vi "Initialize Instrument Engine.vi"(8 "error in (no error)":errorcluster, 9 "Name":string, 11 "Process":refnum<class "Process.lvclass">) -> (0 "error out":errorcluster, 2 "notification":bool, 3 "State Variables":T1)   [LabVIEW 2023, in "Instrument Addon Engine.lvlib"]
uses:
  Instrument Addon Engine.lvlib
  Types/Engine State Variables.ctl
  <vilib>/NI/NI VeriStand Addon Network Comm/Engine/VeriStand Comm.lvclass
  <vilib>/NI/NIVS Inline Async API/_Data Access Engine/Data Access Engine/Types/Write.DVR.ctl
  <vilib>/NI/NIVS Inline Async API/_Data Access Engine/Access Type Classes/Write/Write.lvclass
  <vilib>/NI/NIVS Inline Async API/_Data Access Engine/Data Access Engine/Types/Read.DVR.ctl
  <vilib>/NI/NIVS Inline Async API/_Data Access Engine/Access Type Classes/Read/Read.lvclass
  <vilib>/NI/NIVS Inline Async API/_Data Access Engine/Data Access Engine/Types/ReadWrite.DVR.ctl
  <vilib>/NI/NIVS Inline Async API/_Data Access Engine/Access Type Classes/ReadWrite/ReadWrite.lvclass
  <vilib>/NI/NI VeriStand Addon Network Comm/Engine/VeriStand Comm.lvclass/VeriStand Comm.ctl
  <vilib>/NI/NIVS Inline Async API/_VS Inline Async API/Process/Process.lvclass/Process.ctl
  <vilib>/NI/NIVS Inline Async API/_VS Inline Async API/Error Handling Process/SubVIs/Error.ConvertArray.vi
  Addon Shared/SubVIs/Constants.vi
  <vilib>/Utility/SystemLogging/Write to System Log.vi
  <vilib>/NI/AMC/Create Message Queue.vi
  <vilib>/NI/STM/Connection Manager/TCP/Advanced/TCP Initialize Connection Manager (By Reference).vi
  <vilib>/NI/NIVS Inline Async API/_Data Access Engine/Data Access Engine/Methods/Write.Lookup.vi
  <vilib>/NI/NIVS Inline Async API/_Data Access Engine/Data Access Engine/Methods/Read.Lookup.vi
  <vilib>/NI/NIVS Inline Async API/_Data Access Engine/Data Access Engine/Methods/ReadWrite.Lookup.vi
  <vilib>/NI/NIVS Inline Async API/_Data Access Engine/Data Access Engine/Data Access Engine.lvclass
  Addon Shared/Instrument Addon Shared.lvlib
  <vilib>/NI/NIVS Inline Async API/_VS Inline Async API/Process/Process.lvclass
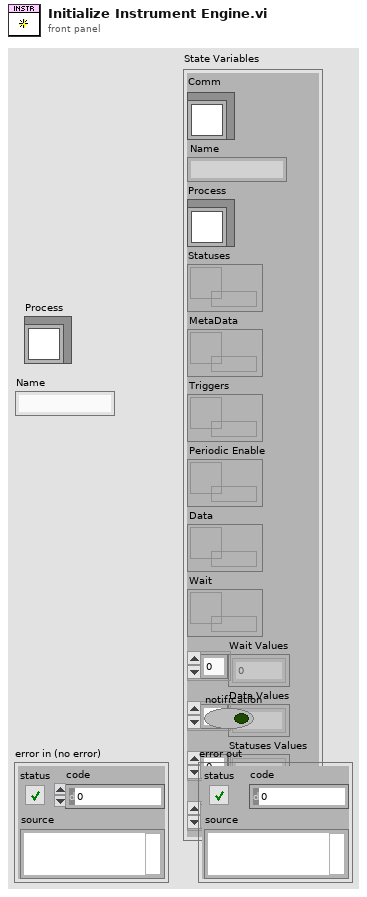
[diagram p1: front panel]
types:
  T1 = typedef "Instrument Addon Engine.lvlib/Engine State Variables.ctl" = cluster{"Comm":refnum<class "VeriStand Comm.lvclass">, "Name":string, "Process":refnum<class "Process.lvclass">, "Statuses":T2, "MetaData":T3, "Triggers":T4, "Periodic Enable":T3, "Data":T2, "Wait":T3, "Wait Values":dbl[], "Data Values":dbl[], "Statuses Values":dbl[], "MetaData Values":dbl[]}
  T2 = typedef "Data Access Engine.lvlib/Data Access Engine.lvclass/Write.DVR.ctl" = refnum<data-value>
  T3 = typedef "Data Access Engine.lvlib/Data Access Engine.lvclass/Read.DVR.ctl" = refnum<data-value>
  T4 = typedef "Data Access Engine.lvlib/Data Access Engine.lvclass/ReadWrite.DVR.ctl" = refnum<data-value>
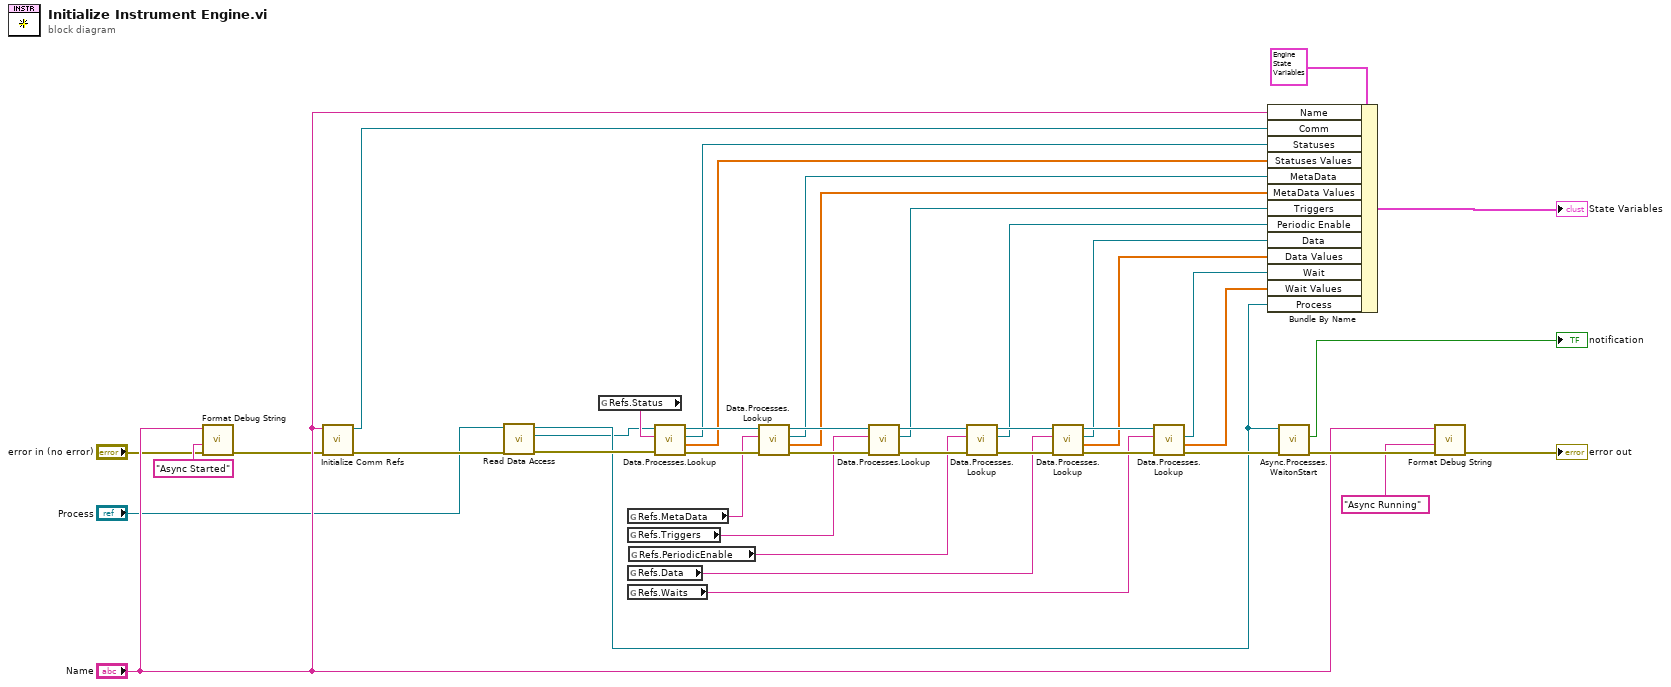
[diagram p0: block diagram]
diagram:
  n1 = call "Format Debug String.vi"("error in (no error)"="error in (no error)", "State"="Async Started" ("string"), "Name"="Name") -> ("error out"=w6:errorcluster)  [unwired: 7 in, 1 out]
  n2 = call <vilib>:"Initialize Comm Refs.vi"("error in (no error)"=w6, "Name"="Name") -> ("error out"=w5:errorcluster, "Comm.lvclass"=w42:refnum<class "VeriStand Comm.lvclass">)  [unwired: 8 in]
  n3 = call <vilib>:"Read Data Access.vi"("error in (no error)"=w5, "Process in"="Process") -> ("error out"=w4:errorcluster, "Data Access"=w1:refnum<class "Data Access Engine.lvclass">, "Process out"=w3:refnum<class "Process.lvclass">)  [unwired: 7 in]
  n4 = global read "Constants.vi" "Refs.Status"() -> (w24:string)
  n5 = global read "Constants.vi" "Refs.MetaData"() -> (w23:string)
  n6 = global read "Constants.vi" "Refs.Triggers"() -> (w21:string)
  n7 = global read "Constants.vi" "Refs.Data"() -> (w19:string)
  n8 = global read "Constants.vi" "Refs.Waits"() -> (w18:string)
  n9 = global read "Constants.vi" "Refs.PeriodicEnable"() -> (w20:string)
  n10 = call-poly <vilib>:"Data.Processes.Lookup.vi"("error in (no error)"=w4, "Name"=w24, "Data Access API in"=w1) -> ("error out"=w25:errorcluster, "Initial Values"=w15:dbl[], "Ref"=w13:T2, "Data Access API out"=w39:refnum<class "Data Access Engine.lvclass">)  [unwired: 5 in]
  n11 = call-poly <vilib>:"Data.Processes.Lookup.vi"("error in (no error)"=w25, "Name"=w23, "Data Access API in"=w39) -> ("error out"=w22:errorcluster, "Initial Values"=w16:dbl[], "Ref"=w26:T3, "Data Access API out"=w38:refnum<class "Data Access Engine.lvclass">)  [unwired: 5 in]
  n12 = call-poly <vilib>:"Data.Processes.Lookup.vi"("error in (no error)"=w22, "Name"=w21, "Data Access API in"=w38) -> ("error out"=w28:errorcluster, "Ref"=w27:T4, "Data Access API out"=w37:refnum<class "Data Access Engine.lvclass">)  [unwired: 5 in, 1 out]
  n13 = call-poly <vilib>:"Data.Processes.Lookup.vi"("error in (no error)"=w28, "Name"=w20, "Data Access API in"=w37) -> ("error out"=w29:errorcluster, "Ref"=w30:T3, "Data Access API out"=w36:refnum<class "Data Access Engine.lvclass">)  [unwired: 5 in, 1 out]
  n14 = call-poly <vilib>:"Data.Processes.Lookup.vi"("error in (no error)"=w29, "Name"=w19, "Data Access API in"=w36) -> ("error out"=w31:errorcluster, "Initial Values"=w14:dbl[], "Ref"=w32:T2, "Data Access API out"=w35:refnum<class "Data Access Engine.lvclass">)  [unwired: 5 in]
  n15 = call-poly <vilib>:"Data.Processes.Lookup.vi"("error in (no error)"=w31, "Name"=w18, "Data Access API in"=w35) -> ("error out"=w34:errorcluster, "Initial Values"=w17:dbl[], "Ref"=w33:T3)  [unwired: 5 in, 1 out]
  n16 = Bundle By Name(cluster=T1 {"Comm"=refnum, "Name"="", "Process"=refnum, "Statuses"=refnum, "MetaData"=refnum, "Triggers"=refnum, "Periodic Enable"=refnum, "Data"=refnum, "Wait"=refnum, "Wait Values"=[], "Data Values"=[], "Statuses Values"=[], "MetaData Values"=[]} ("State Variables"), "Name"="Name", "Comm"=w42, "Statuses"=w13, "Statuses Values"=w15, "MetaData"=w26, "MetaData Values"=w16, "Triggers"=w27, "Periodic Enable"=w30, "Data"=w32, "Data Values"=w14, "Wait"=w33, "Wait Values"=w17, "Process"=w3) -> (→"State Variables":T1)
  n17 = call <vilib>:"Async.Processes.WaitonStart.vi"("error in (no error)"=w34, "Process"=w3) -> ("error out"=w11:errorcluster, "Execute"=→"notification":bool)  [unwired: 7 in, 1 out]
  n18 = call "Format Debug String.vi"("error in (no error)"=w11, "State"="Async Running" ("string"), "Name"="Name") -> ("error out"=→"error out":errorcluster)  [unwired: 7 in, 1 out]
